vi "Read Direction.vi"(8 "error in (no error)":errorcluster, 9 "Direction SEQ":refnum<queue>, 11 "Game Board in":refnum<class "Game Board.lvclass">) -> (0 "error out":errorcluster, 3 "Game Board out":refnum<class "Game Board.lvclass">)   [LabVIEW 2015, in "Game Board.lvclass"]
uses:
  Game Board.lvclass
  Snake/Type Defs/Direction.ctl
  Game Board.lvclass/Game Board.ctl
  Snake/Snake.lvclass/Snake.ctl
  Snake/Snake.lvclass
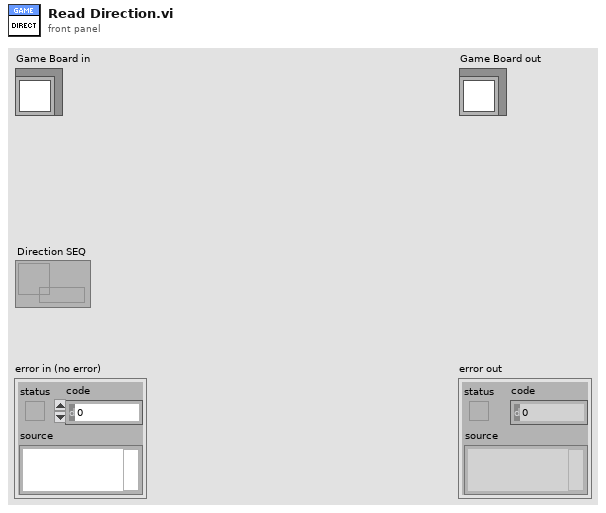
[diagram p1: front panel]
types:
  T1 = typedef "Direction.ctl" = enum16{"Up", "Down", "Left", "Right"}
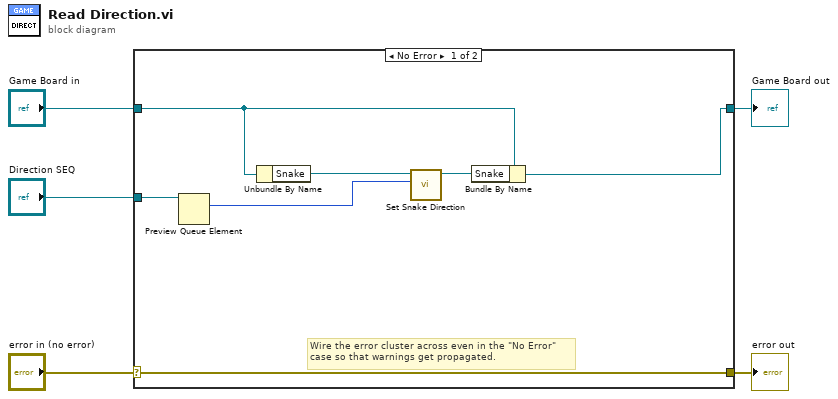
[diagram p0: block diagram]
diagram:
  n1 = case shown="No Error" "error in (no error)" {
    selector: "error in (no error)" -> [w12 w14]
    tunnel: [w12 w14] -> w4
    tunnel: [w8 w13] -> w2
    tunnel: "Game Board in" -> [w9 w13]
    tunnel: "Direction SEQ" -> [w11 _]
    frame No Error {
      # "Wire the error cluster across even in the \"No Error\"\ncase so that warnings get propagated."
      n2 = Preview Queue Element(queue=w11) -> (element=w6:T1)  [unwired: 2 in, 3 out]
      n3 = Unbundle By Name(w9) -> ("Snake"=w10:refnum<class "Snake.lvclass">)
      n4 = call "Set Snake Direction.vi"("Direction"=w6, "Snake in"=w10) -> ("Snake out"=w7:refnum<class "Snake.lvclass">)  [unwired: 8 in, 1 out]
      n5 = Bundle By Name(cluster=w9, "Snake"=w7) -> (w8:refnum<class "Game Board.lvclass">)
    }
    frame Error {
    }
  }
  "error out" <- w4
  "Game Board out" <- w2
